vi "Write Step Result.vi"(8 "error in (no error)":errorcluster, 10 "Pass?":bool, 11 "Step Index":i32) -> (0 "error out":errorcluster)   [LabVIEW 2015, in "UI Handler.lvclass"]
uses:
  UI Handler.lvclass
  UI Handler.lvclass/UI Handler.ctl
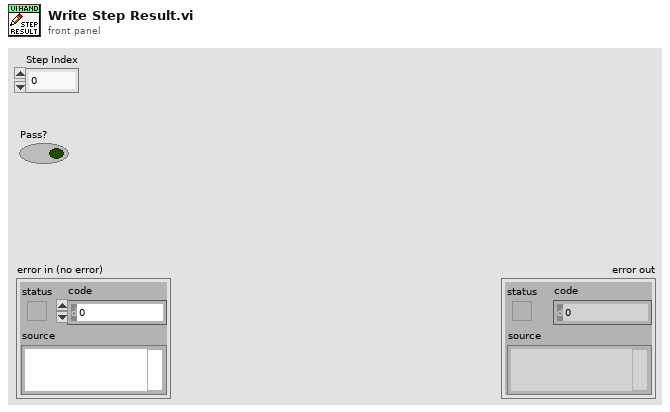
[diagram p1: front panel]
types:
  T1 = typedef "UI Handler.lvclass/Session Handle.ctl" = refnum<data-value>
  T2 = cluster{"Step Index":i32, "disabled index (col)":i32}
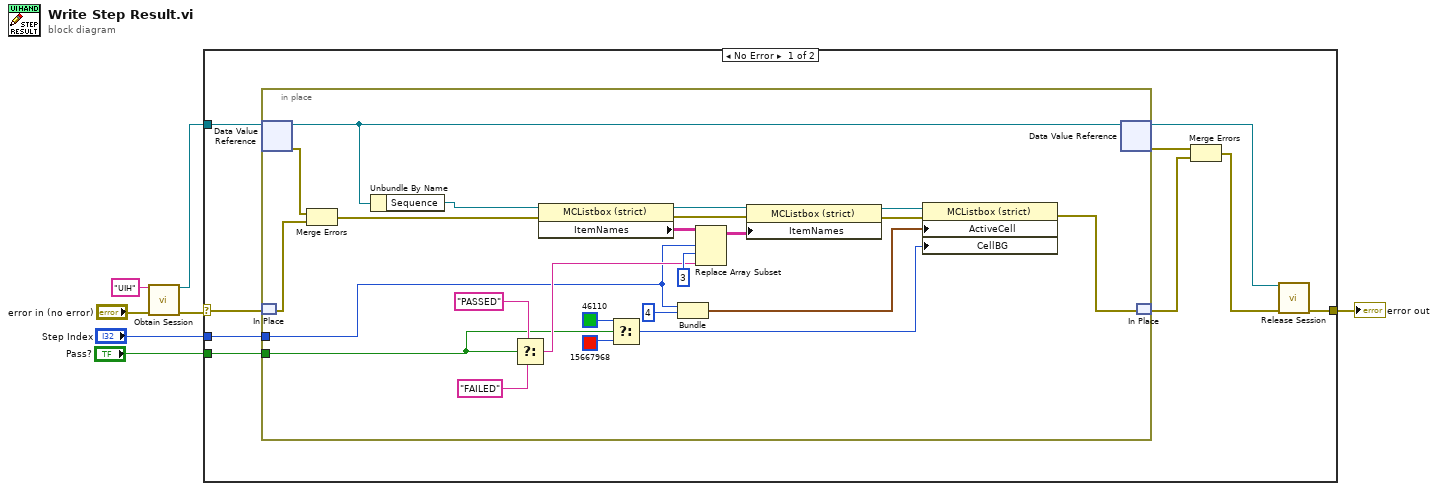
[diagram p0: block diagram]
diagram:
  n1 = call "Obtain Session.vi"("Session  Name ()"="UIH", "error in (no error)"="error in (no error)") -> ("Session Handle"=w3:T1, "error out"=w4:errorcluster)  [unwired: 12 in]
  n2 = case shown="No Error" w4 {
    selector: w4 -> [w13 w40]
    tunnel: w3 -> [w16 _]
    tunnel: [w9 w40] -> w6
    tunnel: "Step Index" -> [w12 _]
    tunnel: "Pass?" -> [w11 _]
    frame No Error {
      n3 = in-place {
        in-place-border: w12 -> [w19]
        in-place-border: w11 -> [w17]
        n4 = in-place-dvr #1(w16) -> (w39:refnum<class "UI Handler.lvclass">, w21:errorcluster)
        n5 = in-place-match #2(w13) -> (w20:errorcluster)
        n6 = Merge Errors(w21, w20) -> (w22:errorcluster)
        n7 = Unbundle By Name(w39) -> ("Sequence"=w23:refnum<vi>)
        n8 = Select(t="PASSED", s=w17, f="FAILED") -> (s? t:f=w34:string)
        n9 = property on="Property Node" class="MCListbox (strict)"(reference=w23, error in=w22) -> (reference out=w30:refnum<vi>, error out=w28:errorcluster, "ItemNames"=w38:string[][])
        n10 = Select(t=u32 46110, s=w17, f=u32 15667968) -> (s? t:f=w25:u32)
        n11 = Bundle("Step Index"=w19, "disabled index (col)"=4) -> (w26:T2)  [unwired: 1 in]
        n12 = Replace Array Subset(array=w38, new element=w34, index (row)=w19, index (col)=3 ("disabled index (col)")) -> (w33:string[][])
        n13 = property on="Property Node" class="MCListbox (strict)"(reference=w30, error in=w28, "ItemNames"=w33) -> (reference out=w29:refnum<vi>, error out=w27:errorcluster)
        n14 = property on="Property Node" class="MCListbox (strict)"(reference=w29, error in=w27, "ActiveCell"=w26, "CellBG"=w25) -> (error out=w18:errorcluster)  [unwired: 1 out]
        n15 = in-place-dvr #1(w39) -> (w8:T1, w14:errorcluster)
        n16 = in-place-match #2(w18) -> (w15:errorcluster)
      }
      n17 = Merge Errors(w14, w15) -> (w10:errorcluster)
      n18 = call "Release Session.vi"("Session Handle"=w8, "error in (no error)"=w10) -> ("error out"=w9:errorcluster)  [unwired: 13 in]
    }
    frame Error {
    }
  }
  "error out" <- w6
